vi "Teleop Gear V.5.0.vi"   [LabVIEW 2016]
uses:
  <vilib>/Rock Robotics/WPI/Solenoid/WPI_SolenoidValue.ctl
  Robot Global Data V.5.0.vi
  <vilib>/Rock Robotics/WPI/Solenoid/WPI_SolenoidSetEnum.vi
types:
  T1 = typedef "WPI_SolenoidValue.ctl" = enum16{"Off", "On", "Forward", "Reverse"}
  T2 = typedef "WPI_ServoDeviceRef.ctl" = cluster{"DeviceStatus":errorcluster, "PWM Channel":T3, "DeadBand":T4}
  T3 = typedef "FPGA_DIOPWMChannel.ctl" = enum8{"PWM 0", "PWM 1", "PWM 2", "PWM 3", "PWM 4", "PWM 5", "PWM 6", "PWM 7", "PWM 8", "PWM 9", "PWM MXP 0", "PWM MXP 1", "PWM MXP 2", "PWM MXP 3", "PWM MXP 4", "PWM MXP 5", "PWM MXP 6", "PWM MXP 7", "PWM MXP 8", "PWM MXP 9", "Invalid"}
  T4 = typedef "WPI_PWMDeadband.ctl" = cluster{"Name":string, "maxPositivePwm":i32, "minPositivePwm":i32, "centerPwm":i32, "maxNegativePwm":i32, "minNegativePwm":i32, "angularRange":u16}
  T5 = typedef "WPI_SolenoidDevRef.ctl" = cluster{"DevStatus":errorcluster, "Pneumatics Control Module":u8, "Forward Solenoid Channel":T6, "Reverse Solenoid Channel":T6}
  T6 = typedef "WPI_SolenoidChannel.ctl" = enum8{"Solenoid 0", "Solenoid 1", "Solenoid 2", "Solenoid 3", "Solenoid 4", "Solenoid 5", "Solenoid 6", "Solenoid 7", "Invalid"}
  T7 = typedef "WPI_MotorControlDeviceRef.ctl" = cluster{"DeviceStatus":errorcluster, "Type":T8, "PWM":cluster{"PWM Channel":T3, "DeadBand":T4}, "CAN":cluster{"Device Number":u8, "SetOutput VI Ref":variant, "GetOutput VI Ref":variant, "Enable VI Ref":variant, "Disable VI Ref":variant, "Data":variant}, "Invert":bool}
  T8 = typedef "WPI_MotorControlType.ctl" = enum16{"PWM", "CAN"}
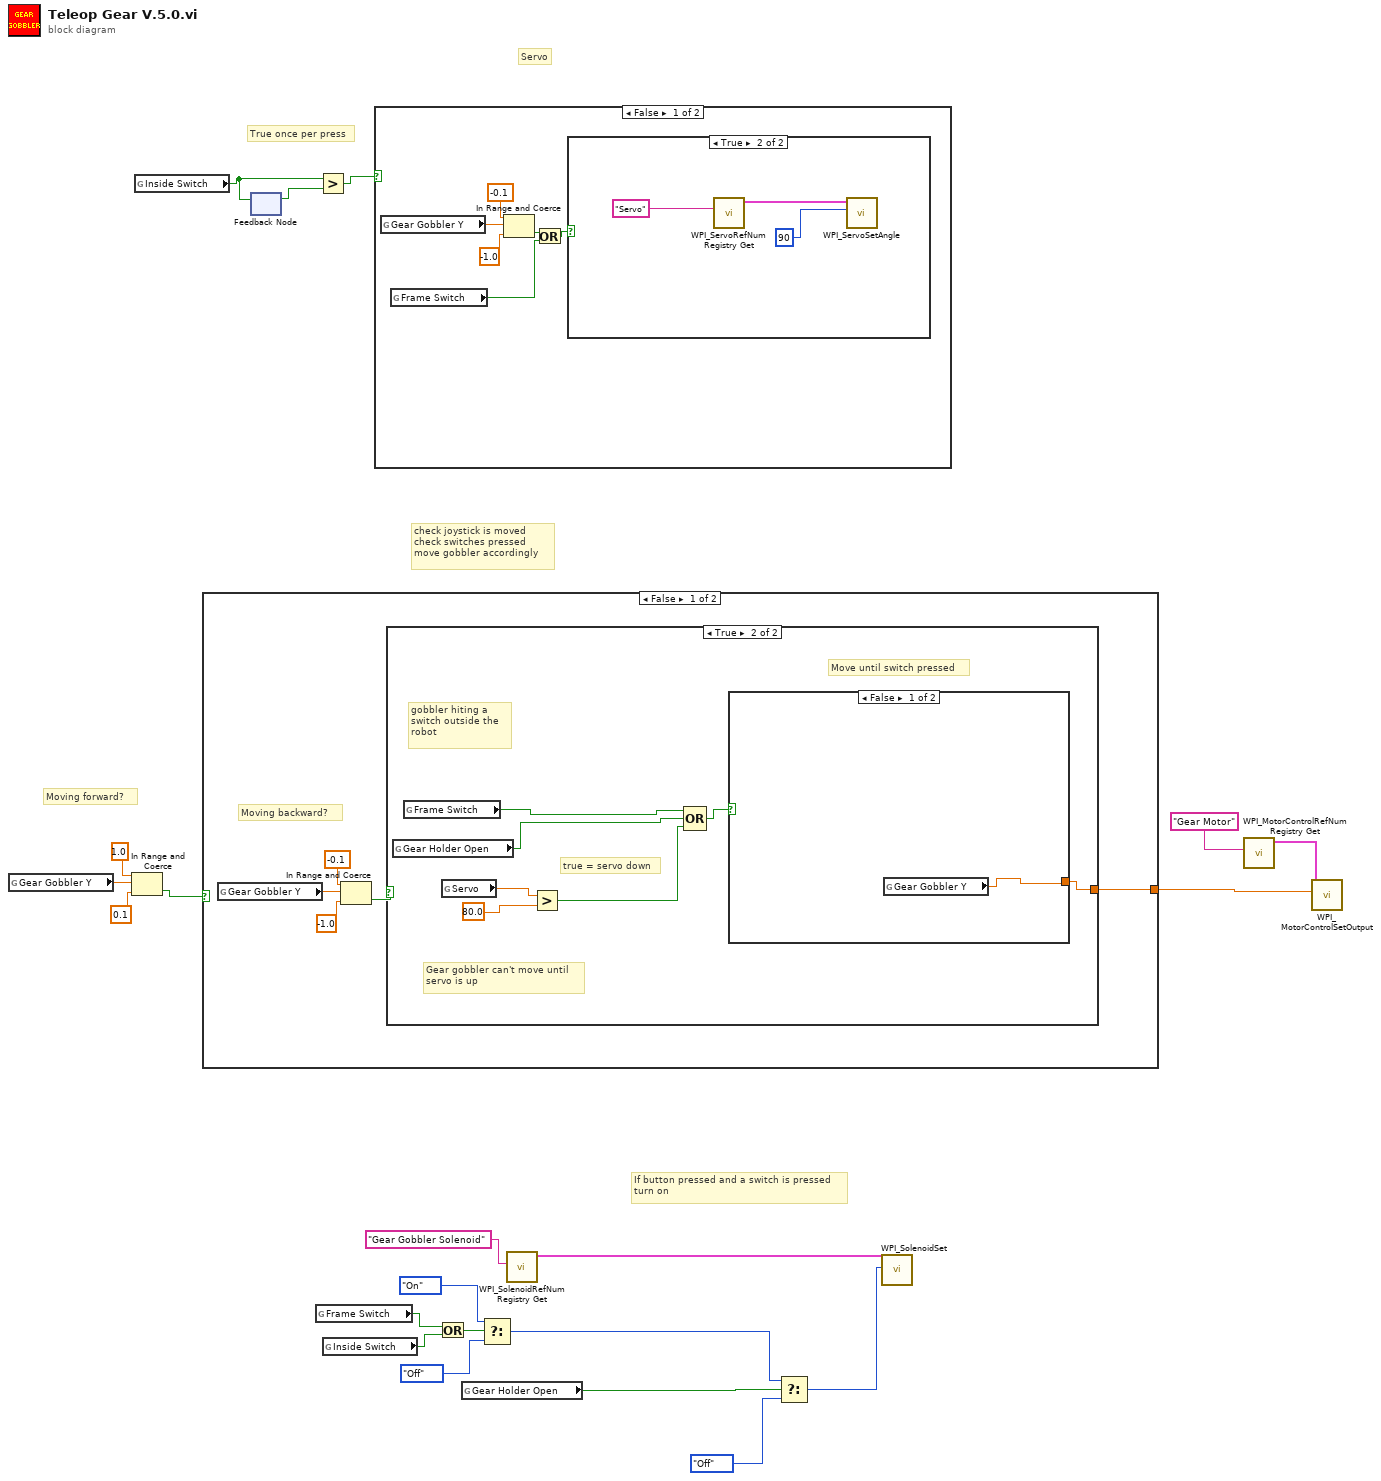
[diagram p0: block diagram]
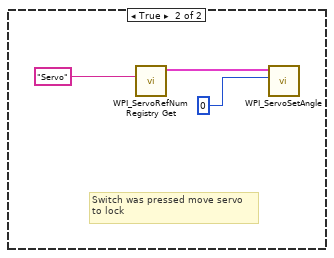
[diagram p3: hidden frame]
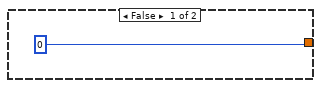
[diagram p4: hidden frame]
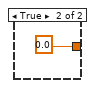
[diagram p5: hidden frame]
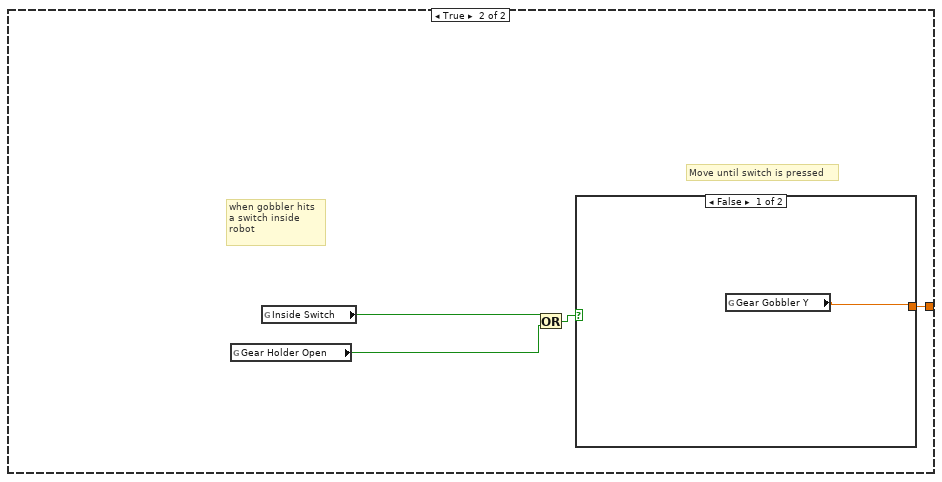
[diagram p6: hidden frame]
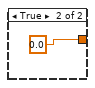
[diagram p7: hidden frame]
diagram:
  # "Servo"
  # "True once per press"
  # "If button pressed and a switch is pressed\nturn on"
  # "check joystick is moved\ncheck switches pressed\nmove gobbler accordingly"
  # "Moving forward?"
  n1 = global read "Robot Global Data V.5.0.vi" "Gear Gobbler Y"() -> (w13:dbl)
  n2 = In Range and Coerce(upper limit=1.0, x=w13, lower limit=0.1) -> (In Range?=w10:bool)  [unwired: 1 out]
  n3 = global read "Robot Global Data V.5.0.vi" "Inside Switch"() -> (w2:bool)
  n4 = case shown="False" w10 {
    tunnel: [w22 w40] -> w19
    frame False {
      # "Moving backward?"
      n5 = global read "Robot Global Data V.5.0.vi" "Gear Gobbler Y"() -> (w26:dbl)
      n6 = In Range and Coerce(upper limit=-0.1, x=w26, lower limit=-1.0) -> (In Range?=w23:bool)  [unwired: 1 out]
      n7 = case shown="True" w23 {
        tunnel: [0 w34] -> w22
        frame False {
        }
        frame True {
          # "true = servo down"
          # "Gear gobbler can't move until\nservo is up"
          # "gobbler hiting a \nswitch outside the \nrobot"
          # "Move until switch pressed"
          n8 = global read "Robot Global Data V.5.0.vi" "Gear Holder Open"() -> (w30:bool)
          n9 = global read "Robot Global Data V.5.0.vi" "Frame Switch"() -> (w31:bool)
          n10 = global read "Robot Global Data V.5.0.vi" "Servo"() -> (w33:dbl)
          n11 = Greater?(x=w33, y=80.0) -> (0:w29:bool)
          n12 = Compound Arithmetic op=OR(w31, w30, w29) -> (w28:bool)
          n13 = case shown="False" w28 {
            tunnel: [w35 0.0] -> w34
            frame False {
              n14 = global read "Robot Global Data V.5.0.vi" "Gear Gobbler Y"() -> (w35:dbl)
            }
            frame True {
            }
          }
        }
      }
    }
    frame True {
      # "when gobbler hits\na switch inside \nrobot"
      # "Move until switch is pressed"
      n15 = global read "Robot Global Data V.5.0.vi" "Gear Holder Open"() -> (w37:bool)
      n16 = global read "Robot Global Data V.5.0.vi" "Inside Switch"() -> (w38:bool)
      n17 = Or(x=w38, y=w37) -> (x .or. y?=w39:bool)
      n18 = case shown="False" w39 {
        tunnel: [w41 0.0] -> w40
        frame False {
          n19 = global read "Robot Global Data V.5.0.vi" "Gear Gobbler Y"() -> (w41:dbl)
        }
        frame True {
        }
      }
    }
  }
  n20 = feedback #1() -> (w3:bool)  [unwired: 1 in]
  n21 = feedback-in #1(w2) -> ()
  n22 = global read "Robot Global Data V.5.0.vi" "Frame Switch"() -> (w8:bool)
  n23 = Greater?(x=w2, y=w3) -> (0:w1:bool)
  n24 = global read "Robot Global Data V.5.0.vi" "Inside Switch"() -> (w9:bool)
  n25 = case shown="False" w1 {
    frame False {
      n26 = global read "Robot Global Data V.5.0.vi" "Gear Gobbler Y"() -> (w48:dbl)
      n27 = global read "Robot Global Data V.5.0.vi" "Frame Switch"() -> (w43:bool)
      n28 = In Range and Coerce(upper limit=-0.1, x=w48, lower limit=-1.0) -> (In Range?=w45:bool)  [unwired: 1 out]
      n29 = Or(x=w45, y=w43) -> (x .or. y?=w44:bool)
      n30 = case shown="True" w44 {
        frame False {
        }
        frame True {
          n31 = call <vilib>:"WPI_ServoRefNum Registry Get.vi"("refnum name"="Servo") -> ("ServoDeviceRef"=w50:T2)  [unwired: 9 in, 1 out]
          n32 = call <vilib>:"WPI_ServoSetAngle.vi"("Angle"=90, "ServoDeviceRef"=w50) -> ()  [unwired: 8 in, 2 out]
        }
      }
    }
    frame True {
      # "Switch was pressed move servo\nto lock"
      n33 = call <vilib>:"WPI_ServoRefNum Registry Get.vi"("refnum name"="Servo") -> ("ServoDeviceRef"=w53:T2)  [unwired: 9 in, 1 out]
      n34 = call <vilib>:"WPI_ServoSetAngle.vi"("Angle"=0, "ServoDeviceRef"=w53) -> ()  [unwired: 8 in, 2 out]
    }
  }
  n35 = Or(x=w8, y=w9) -> (x .or. y?=w7:bool)
  n36 = global read "Robot Global Data V.5.0.vi" "Gear Holder Open"() -> (w14:bool)
  n37 = Select(t=WPI_SolenoidValue."On" ("Value"), s=w7, f=WPI_SolenoidValue."Off" ("Value")) -> (s? t:f=w4:T1)
  n38 = call <vilib>:"WPI_SolenoidRefNum Registry Get.vi"("refnum name"="Gear Gobbler Solenoid") -> ("SolenoidDevRef"=w17:T5)  [unwired: 9 in, 1 out]
  n39 = Select(t=w4, s=w14, f=WPI_SolenoidValue."Off" ("Value")) -> (s? t:f=w15:T1)
  n40 = call-poly <vilib>:"WPI_SolenoidSet.vi"("Value"=w15, "SolenoidDevRef"=w17) -> ()  [unwired: 8 in, 2 out]
  n41 = call <vilib>:"WPI_MotorControlRefNum Registry Get.vi"("refnum name"="Gear Motor") -> ("MotorControlDevRef"=w20:T7)  [unwired: 9 in, 1 out]
  n42 = call <vilib>:"WPI_MotorControlSetOutput.vi"("Output"=w19, "MotorControlDevRef"=w20) -> ()  [unwired: 7 in, 3 out]
